vi "Template Message Loop.vi"(8 "error in (no error)":errorcluster, 9 "Data Queue":refnum<queue>, 10 "Data Notifier":refnum<notifier>, 11 "Message Queues":T1) -> (0 "error out":errorcluster)   [LabVIEW 2015, in "Loop Library Template.lvlib"]
uses:
  Loop Library Template.lvlib
  support/Message Queue/All Message Queues.ctl
  support/Message Queue/Message Cluster.ctl
  Template Configuration.ctl
  Template State.ctl
  Template Loop State.ctl
  <vilib>/Utility/error.llb/Error Cluster From Error Code.vi
  <vilib>/ErrorRing/Error Ring.xnode
  support/Message Queue/Message Queue.lvlib
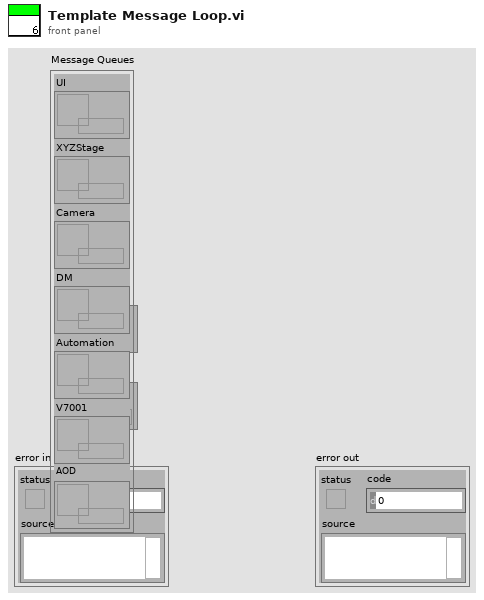
[diagram p1: front panel]
types:
  T1 = typedef "Message Queue.lvlib/All Message Queues.ctl" = cluster{"UI":refnum<queue>, "XYZStage":refnum<queue>, "Camera":refnum<queue>, "DM":refnum<queue>, "Automation":refnum<queue>, "V7001":refnum<queue>, "AOD":refnum<queue>}
  T2 = typedef "Loop Library Template.lvlib/Template State.ctl" = cluster{"<Template> State":T3, "Handle out":u32}
  T3 = typedef "Loop Library Template.lvlib/Template Loop State.ctl" = enum16{"Idle"}
  T4 = typedef "Loop Library Template.lvlib/Template Configuration.ctl" = cluster{" Index":u32}
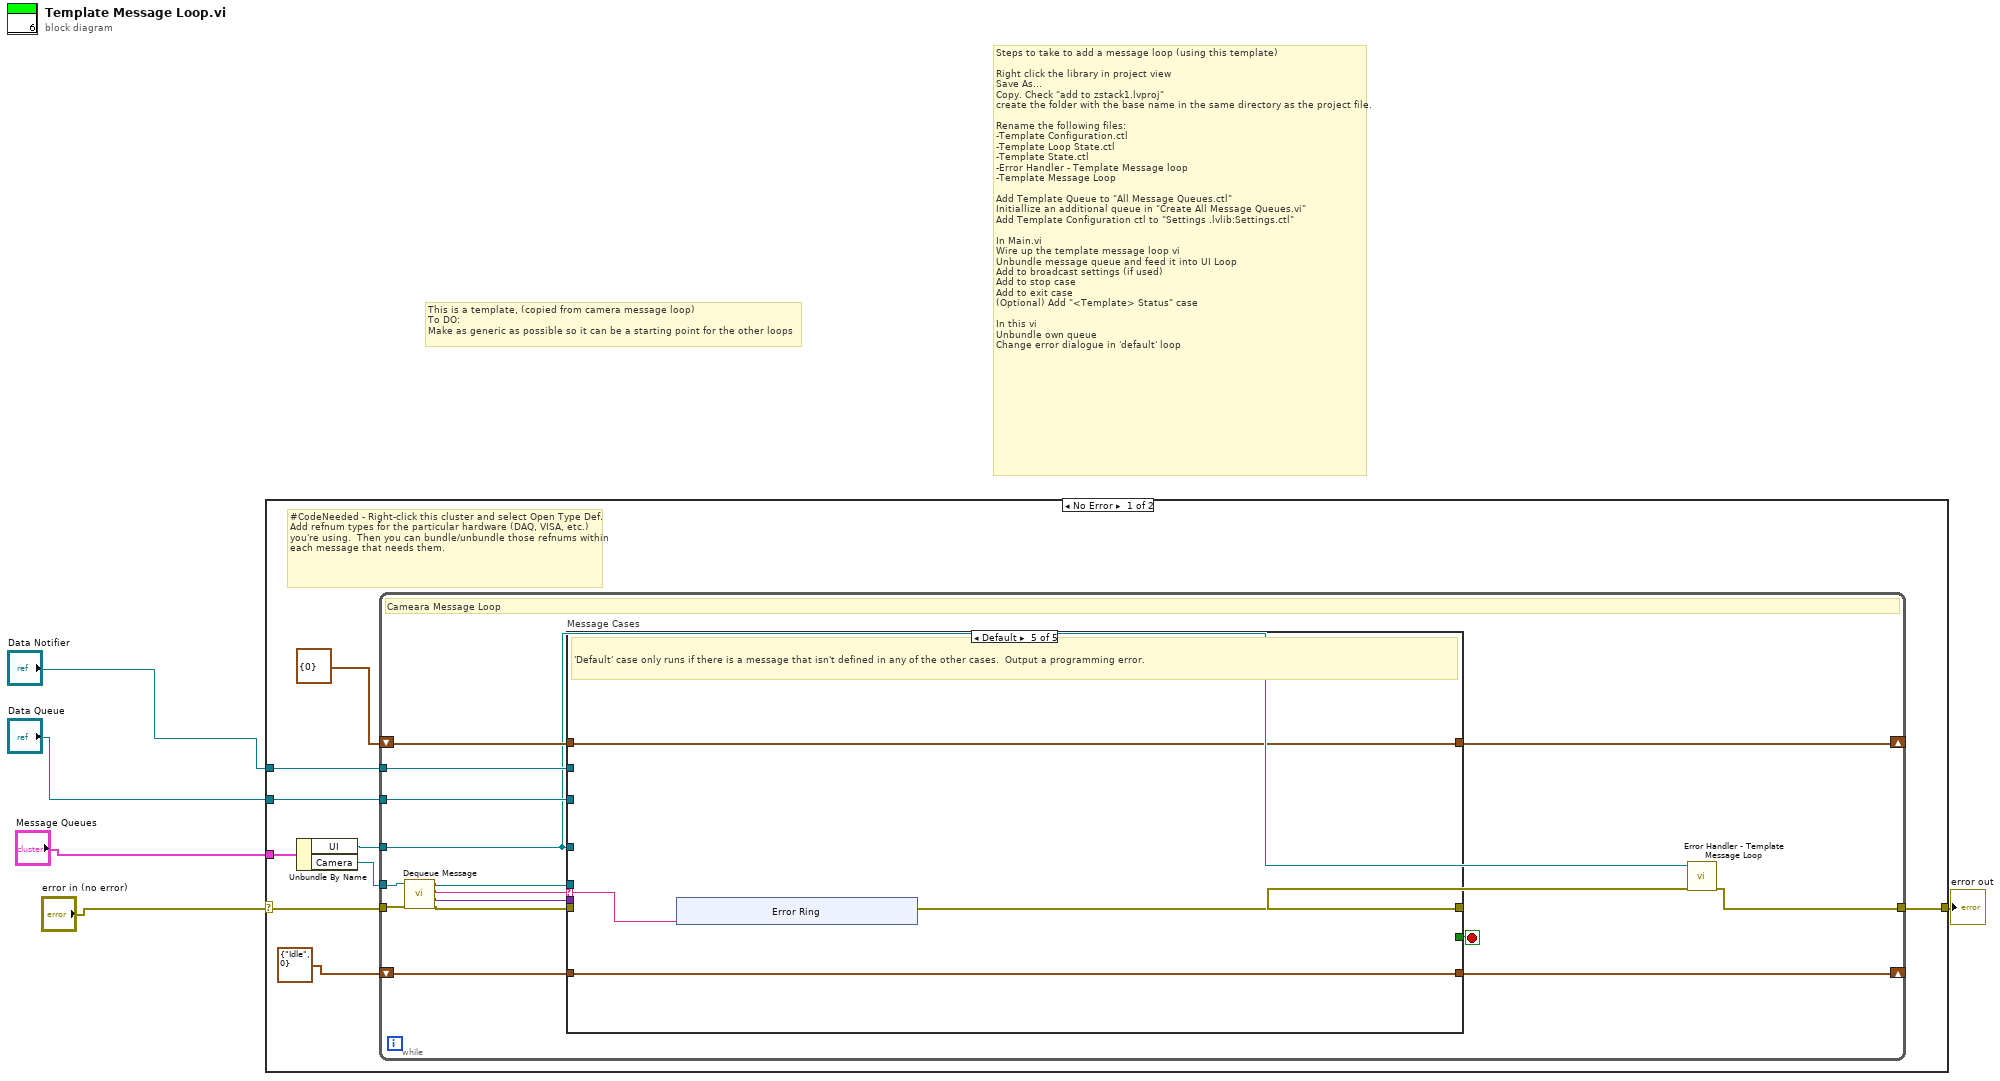
[diagram p0: block diagram]
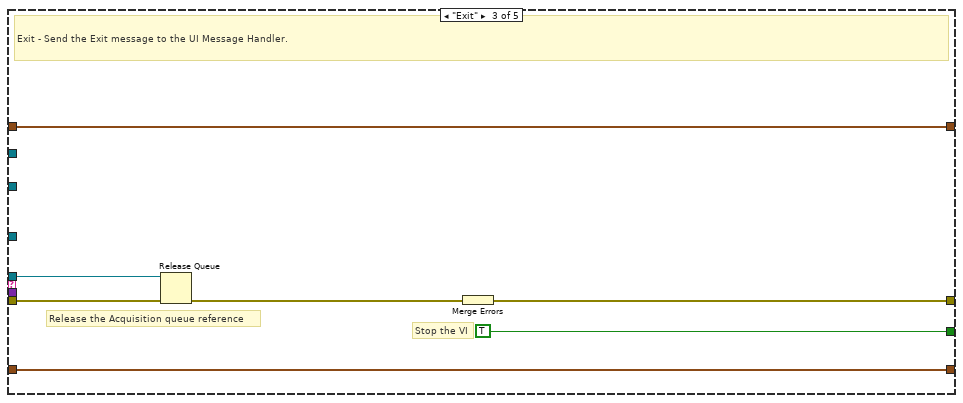
[diagram p4: hidden frame]
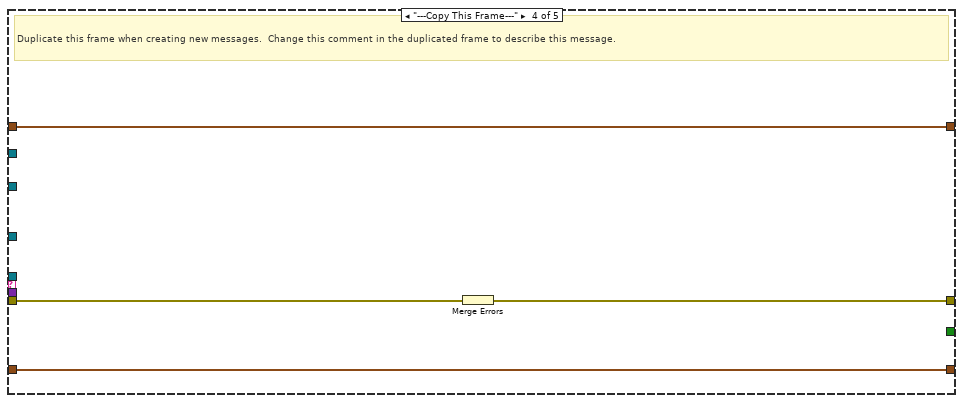
[diagram p5: hidden frame]
diagram:
  # "Steps to take to add a message loop (using this template)\n\nRight click the library in project view\nSave As...\nCopy. Check \"add to zstack1.lvproj\"\ncreate the folder with the base name in the same directory as the project file.\n\nRename the following files:\n-Template Configuration.ctl\n-Template Loop State.ctl\n-Template State.ctl\n-Error Handler - Template Message loop\n-Template Message Loop\n\nAdd Template Queue to \"All Message Queues.ctl\"\nInitiallize an additional queue in \"Create All Message Queues.vi\"\nAdd Template Configuration ctl to \"Settings .lvlib:Settings.ctl\"\n\nIn Main.vi\nWire up the template message loop vi\nUnbundle message queue and feed it into UI Loop\nAdd to broadcast settings (if used)\nAdd to stop case\nAdd to exit case\n(Optional) Add \"<Template> Status\" case\n\nIn this vi\nUnbundle own queue\nChange error dialogue in 'default' loop"
  # "This is a template, (copied from camera message loop)\nTo DO:\nMake as generic as possible so it can be a starting point for the other loops"
  n1 = case shown="No Error" "error in (no error)" {
    selector: "error in (no error)" -> [w11 w59]
    tunnel: "Message Queues" -> [w14 _]
    tunnel: [w12 w59] -> w5
    tunnel: "Data Notifier" -> [w9 _]
    tunnel: "Data Queue" -> [w8 _]
    frame No Error {
      # "#CodeNeeded - Right-click this cluster and select Open Type Def.  Add refnum types for the particular hardware (DAQ, VISA, etc.) you're using.  Then you can bundle/unbundle those refnums within each message that needs them."
      n2 = Unbundle By Name(w14) -> ("UI"=w10:refnum<queue>, "Camera"=w13:refnum<queue>)
      n3 = while {
        tunnel: w13 -> [w23]
        shift-right: [w29] -> _
        shift-left: T4 {" Index"=0} ("Hardware Configuration") -> [w30]
        tunnel: w10 -> [w15]
        tunnel: w9 -> [w27]
        tunnel: w8 -> [w26]
        shift-right: [w24] -> _
        shift-left: T2 {"<Template> State"=enum."Idle", "Handle out"=0} ("Cluster") -> [w25]
        tunnel: w11 -> [w22]
        tunnel: [w17] -> w12
        stop <- w28 stop-if-true
        # "Cameara Message Loop"
        n4 = call "Dequeue Message.vi"("error in (no error)"=w22, "Message Queue"=w23) -> ("error out"=w18:errorcluster, "Message Data"=w19:variant, "Message"=w20:string, "dup Message Queue"=w21:refnum<queue>)  [unwired: 6 in]
        n5 = case "Message Cases" shown="Default" w20 {
          selector: w20 -> [_ _ _ _ w48]
          tunnel: w21 -> [_ _ w38 _ _]
          tunnel: w18 -> [w33 w36 w40 w47 _]
          tunnel: [w33 w36 w42 w45 w49] -> w16
          tunnel: w30 -> [w31 w35 w41 w46 w51]
          tunnel: [w31 w35 w41 w46 w51] -> w29
          tunnel: [_ _ TRUE _ _] -> w28
          tunnel: w19 -> [_ _ _ _ _]
          tunnel: w15 -> [_ _ _ _ _]
          tunnel: w27 -> [_ _ _ _ _]
          tunnel: w26 -> [_ _ _ _ _]
          tunnel: w25 -> [w32 w34 w37 w44 w50]
          tunnel: [w32 w34 w37 w44 w50] -> w24
          frame "Initialize" {
            # "Initialize  - Initialize is currently a no-op.  The hardware initialization takes place in the 'Start' message."
          }
          frame "Stop" {
          }
          frame "Exit" {
            # "Release the Acquisition queue reference"
            # "Stop the VI"
            # "Exit - Send the Exit message to the UI Message Handler."
            n6 = Release Queue(queue=w38, error in (no error)=w40) -> (error out=w39:errorcluster)  [unwired: 1 in, 2 out]
            n7 = Merge Errors(w39) -> (w42:errorcluster)
          }
          frame "---Copy This Frame---" {
            # "Duplicate this frame when creating new messages.  Change this comment in the duplicated frame to describe this message."
            n8 = Merge Errors(w47) -> (w45:errorcluster)
          }
          frame Default {
            # "'Default' case only runs if there is a message that isn't defined in any of the other cases.  Output a programming error."
            n9 = xnode "Error Ring"("parameter 0"=w48) -> ("error out"=w49:errorcluster)
          }
        }
        n10 = call "Error Handler - Template Message Loop.vi"("error in (no error)"=w16, "Message Queue"=w15) -> ("dup error in"=w17:errorcluster)  [unwired: 8 in, 1 out]
      }
    }
    frame Error {
    }
  }
  "error out" <- w5
